vi "TEST_bench_hyst_sat_drift_parallel_fxp_16_5.vi"() -> ()   [LabVIEW 2017]
uses:
  UnitTests/fpga_harnesses/Sat_Hyst_TestCase/hyst_sat_drift_parallel_input_data.ctl
  <vilib>/Platform/TimedLoop/XDataNode/timing_clust.ctl
  <vilib>/Platform/TimedLoop/XDataNode/nitl_modes.ctl
  <vilib>/Platform/TimedLoop/XDataNode/wakeup.ctl
  <vilib>/rvi/Emulation/niFpgaSctlEmulationGetInTimedLoop.vi
  <vilib>/rvi/Emulation/niFpgaEmulationReportErrorSimple.vi
  <vilib>/rvi/Emulation/niFpgaGetClockAttributes.vi
  <vilib>/rvi/Emulation/niFpgaCriticalErrorInLSC.vi
  <vilib>/rvi/Memory/Memory_Emulation/nirvimemoryFastEmulation.vi
  <vilib>/rvi/Memory/Memory_Emulation/nirvimemoryEmulation.vi
  <vilib>/rvi/Emulation/niFpgaEmulationIsFPGAContextNoSignature.vi
  <vilib>/rvi/DataTransferAndStorage/Container/Common/niFpgaContainerGetUniqueNameForEmu.vi
  <vilib>/rvi/Emulation/niFpgaProcessEmulError.vi
  <vilib>/rvi/errors/nirviReportUnexpectedCaseInternalError (U32).vi
  <vilib>/Platform/TimedLoop/XDataNode/XDataNode.xnode
  <vilib>/rvi/DataTransferAndStorage/Container/XNode/niFpgaContainer.xnode
  <vilib>/Platform/TimedLoop/XDataNode/XDNodeRunTimeDep.lvlib
  UnitTests/fpga_harnesses/Sat_Hyst_TestCase/Sat_Hyst_TestCase.lvclass
panel:
  out "load-ticks":u32
  in  "input cluster":T1
  out "H_of_uk":fxp<+/-,32,10>[](array[numeric])
  in  "uk":sgl[](array[numeric]) format="%#_13g"
  in  "numIter":i32
  in  "y_vec_in":fxp<+/-,16,5>[](array[numeric])=[0.0, 0.0, 0.0, 0.0, 0.0, 0.0, 0.0]
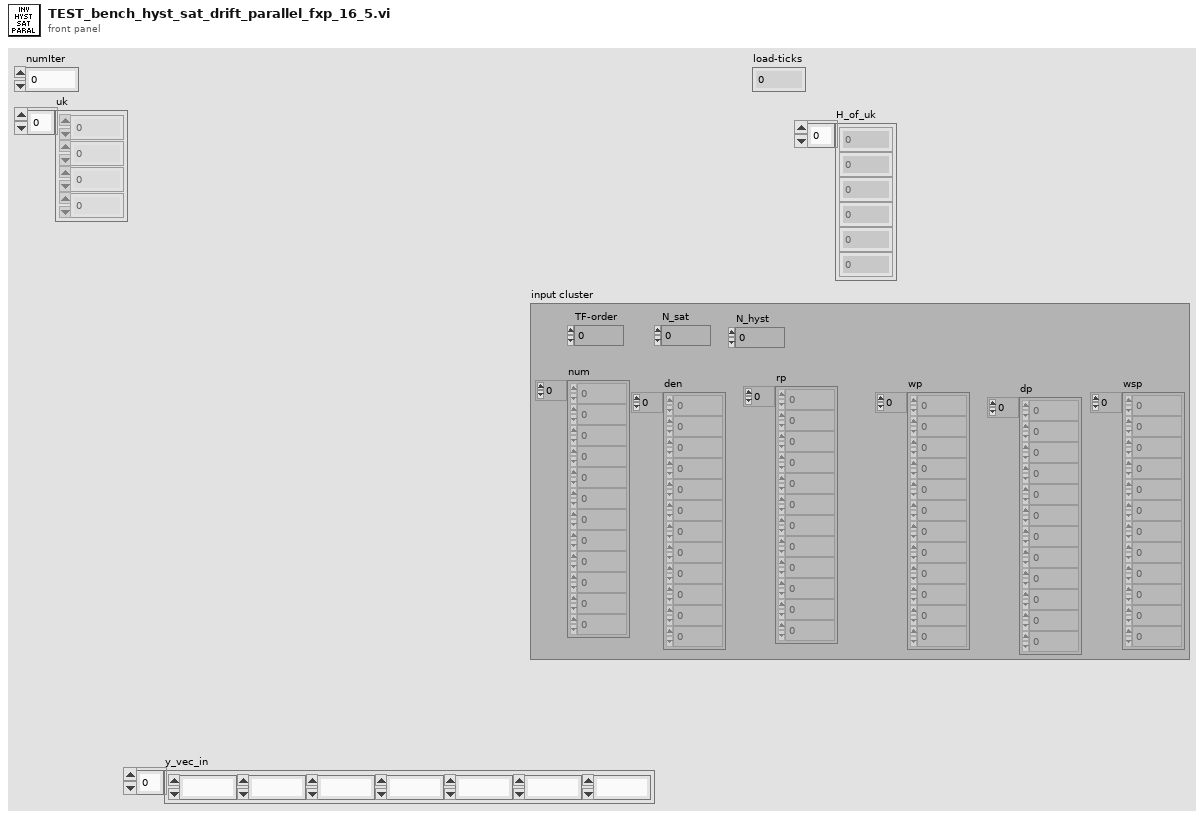
[diagram p1: front panel]
types:
  T1 = typedef "Sat_Hyst_TestCase.lvclass/hyst_sat_drift_parallel_input_data.ctl" = cluster{"TF-order":i32, "N_sat":i32, "N_hyst":i32, "num":sgl[], "wsp":fxp<+/-,16,5>[], "dp":fxp<+/-,16,5>[], "rp":fxp<+/-,16,5>[], "wp":fxp<+/-,16,5>[], "den":sgl[]}
  T2 = typedef "XDNodeRunTimeDep.lvlib/timing_clust.ctl" = cluster{"Expected End [f-1]":u64, "Actual End [f-1]":u64, "Finished Late? [f-1]":bool, "Expected End [i-1]":u64, "Actual End [i-1]":u64, "Finished Late? [i-1]":bool, "Expected Start [i]":u64, "Actual Start [i]":u64, "Expected Start [f]":u64, "Actual Start [f]":u64, "Source Name":string, "Structure Name":string, "Period":i64, "Deadline":i64, "Offset":i64, "Start":i64, "Priority":i32, "Timeout":i32, "Mode":T3, "Wakeup Reason":T4, "Error":errorcluster, "Source Type":string, "Secondary Source Type":string, "Global End Time":u64, "Global Start Time":u64, "Frame Duration":u64, "Iteration Duration":u64, "Assigned CPU":i32, "I/O Scan Engine Mode":u32}
  T3 = typedef "XDNodeRunTimeDep.lvlib/nitl_modes.ctl" = enum32{"No Change", "Process missed periods, maintain original phase", "Discard missed periods, maintain original phase", "Process missed periods, ignore original phase", "Discard missed periods, ignore original phase"}
  T4 = typedef "XDNodeRunTimeDep.lvlib/wakeup.ctl" = enum32{"Normal", "Aborted", "Asynchronous wakeup", "Timing source error", "Timed loop error", "Timeout"}
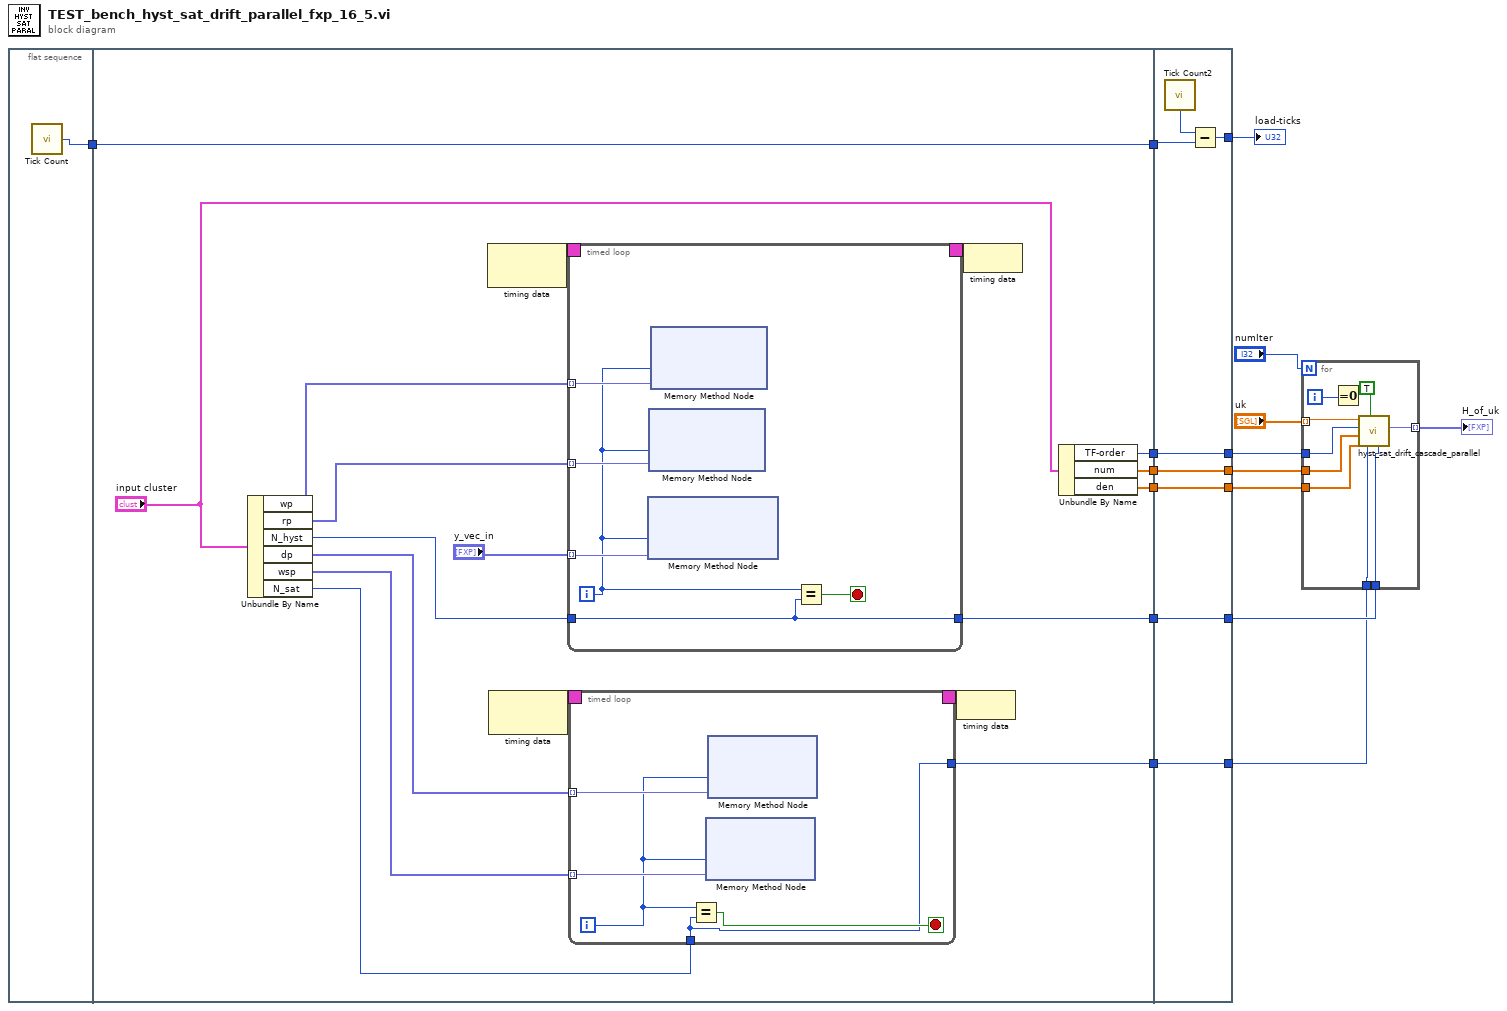
[diagram p0: block diagram]
diagram:
  n1 = flat-sequence {
    tunnel: [w17] -> w2
    tunnel: [w30] -> w8
    tunnel: [w29] -> w7
    tunnel: [w22] -> w6
    tunnel: [w21] -> w5
    tunnel: [w20] -> w4
    tunnel: [w18] -> w3
    tunnel: w2 -> [w18]
    tunnel: [w58] -> w9
    tunnel: [w59] -> w10
    tunnel: [w60] -> w11
    tunnel: [w61] -> w12
    tunnel: [w62] -> w13
    tunnel: w8 -> [w62]
    tunnel: w7 -> [w61]
    tunnel: w6 -> [w60]
    tunnel: w5 -> [w59]
    tunnel: w4 -> [w58]
    tunnel: w3 -> [w56]
    tunnel: [w55] -> w1
    frame #0 {
      n2 = call "Tick Count"() -> ("Tick Count(Ticks)"=w17:u32)
    }
    frame #1 {
      n3 = Unbundle By Name("input cluster") -> ("wp"=w28:fxp<+/-,16,5>[], "rp"=w27:fxp<+/-,16,5>[], "N_hyst"=w26:i32, "dp"=w25:fxp<+/-,16,5>[], "wsp"=w24:fxp<+/-,16,5>[], "N_sat"=w19:i32)
      n4 = node-c288() -> (w35:T2)  [unwired: 1 in]
      n5 = node-c288() -> (w33:T2)  [unwired: 1 in]
      n6 = timed-loop {
        timing: w35 -> [_]
        timing-out: [_] -> w34
        tunnel: w28 -> [w49] mode=indexing
        tunnel: w27 -> [w47] mode=indexing
        tunnel: "y_vec_in" -> [w48] mode=indexing
        tunnel: w26 -> [w46]
        tunnel: [w46] -> w30
        i -> [w45]
        stop <- w50 stop-if-true
        n7 = xnode ("Memory Method Node")("Address"=w45, "Data"=w48) -> ()  [unwired: 1 in, 1 out]
        n8 = xnode ("Memory Method Node")("Address"=w45, "Data"=w47) -> ()  [unwired: 1 in, 1 out]
        n9 = xnode ("Memory Method Node")("Address"=w45, "Data"=w49) -> ()  [unwired: 1 in, 1 out]
        n10 = Equal?(x=w45, y=w46) -> (x = y?=w50:bool)
      }
      n11 = timed-loop {
        timing: w33 -> [_]
        timing-out: [_] -> w32
        tunnel: w25 -> [w40] mode=indexing
        tunnel: w24 -> [w39] mode=indexing
        tunnel: w19 -> [w36]
        tunnel: [w36] -> w29
        i -> [w37]
        stop <- w38 stop-if-true
        n12 = Equal?(x=w37, y=w36) -> (x = y?=w38:bool)
        n13 = xnode ("Memory Method Node")("Address"=w37, "Data"=w39) -> ()  [unwired: 1 in, 1 out]
        n14 = xnode ("Memory Method Node")("Address"=w37, "Data"=w40) -> ()  [unwired: 1 in, 1 out]
      }
      n15 = node-c288(w32) -> ()
      n16 = node-c288(w34) -> ()
      n17 = Unbundle By Name("input cluster") -> ("TF-order"=w22:i32, "num"=w21:sgl[], "den"=w20:sgl[])
    }
    frame #2 {
      n18 = call "Tick Count2"() -> ("Tick Count(Ticks)"=w57:u32)
      n19 = Subtract(x=w57, y=w56) -> (x-y=w55:u32)
    }
  }
  n20 = for {
    N: "numIter" -> [_]
    tunnel: "uk" -> [w68] mode=indexing
    tunnel: [w70] -> w14 mode=indexing
    tunnel: w13 -> [w64]
    tunnel: w12 -> [w63]
    tunnel: w11 -> [w67]
    tunnel: w10 -> [w66]
    tunnel: w9 -> [w65]
    i -> [w71]
    n21 = Equal To 0?(x=w71) -> ()  [unwired: 1 out]
    n22 = call "hyst_sat_drift_cascade_parallel.vi"("N_hyst"=w64, "N_sat"=w63, "parallel_inv"=TRUE, "Den"=w65, "Num"=w66, "TF Order"=w67, "u_k (un saturated)"=w68) -> ("Hinv(uk)"=w70:fxp<+/-,32,10>)  [unwired: 4 in]
  }
  "H_of_uk" <- w14
  "load-ticks" <- w1
